vi "ChuongTrinhLabVIEW.vi"() -> ()   [LabVIEW 2020]
uses:
  <vilib>/MakerHub/LINX/Public/Peripherals/Analog/Analog Read 1 Chan.vi
  <vilib>/MakerHub/LINX/Public/Peripherals/PWM/PWM Set Duty Cycle 1 Chan.vi
  <vilib>/MakerHub/LINX/Public/Peripherals/Analog/Analog Read N Chans.vi
  <vilib>/MakerHub/LINX/Private/Local IO/LinxAnalogRead.vi
  <vilib>/MakerHub/LINX/Public/Utilities/Check Channel.vi
  <vilib>/MakerHub/LINX/Public/Utilities/Open Serial.vi
  <vilib>/addons/control/pid/pid.llb/PID Gain Schedule (DBL).vi
  <vilib>/addons/control/pid/pid.llb/PID (DBL).vi
  <vilib>/MakerHub/LINX/Private/Utilties/Generate Error.vi
  <vilib>/MakerHub/LINX/Public/Peripherals/PWM/PWM Set Duty Cycle N Chans.vi
  <vilib>/MakerHub/LINX/LMH-LINX.lvlib
  <vilib>/addons/control/pid/NI_PID_pid.lvlib
panel:
  in  "Tab Control 3":enum32{"Page 1"}(tab)
  in  "Bang Thong So":string[][](table)
  out "Thong so":T1(graph)
  out "Cam bien khi gas":dbl
  out "nhiet do":dbl(slide) scale=0.0..100.0
  out "Do am":dbl(slide) scale=0.0..100.0
  out "?":dbl
  out "?":dbl
  out "CANH BAO MUA":string
  out "CANH BAO KHI GAS":string
  in  "Tab Control 2":enum32{"PID"}(tab)
  in  "PID gain schedule":T2(array[cluster])=[{"PID gains"={"proportional gain (Kc)"=1.0, "integral time (Ti, min)"=0.01, "derivative time (Td, min)"=0.0}, "max value"=100.0}] {"max value" format="%.2f"; "PID gains"."derivative time (Td, min)" format="%.3f"; "PID gains"."integral time (Ti, min)" format="%.3f"; "PID gains"."proportional gain (Kc)" format="%.3f"}
  out "PID":T3(graph)
  in  "Set point":dbl
  in  "Tab Control":enum32{"Control"}(tab)
  in  "livingRoom":bool
  in  "Control DOOR":bool
  out "State Door":string
  in  "BedRoom":bool
  in  "kitchen":bool
  in  "Control Cua Cuon":bool
  in  "Control Dan Phoi":bool
  out "State Cua Cuon":string
  out "State Dan Phoi":string
  in  "Serial Port":refnum<visa-resource-name>="N/A"
  in  "?":bool
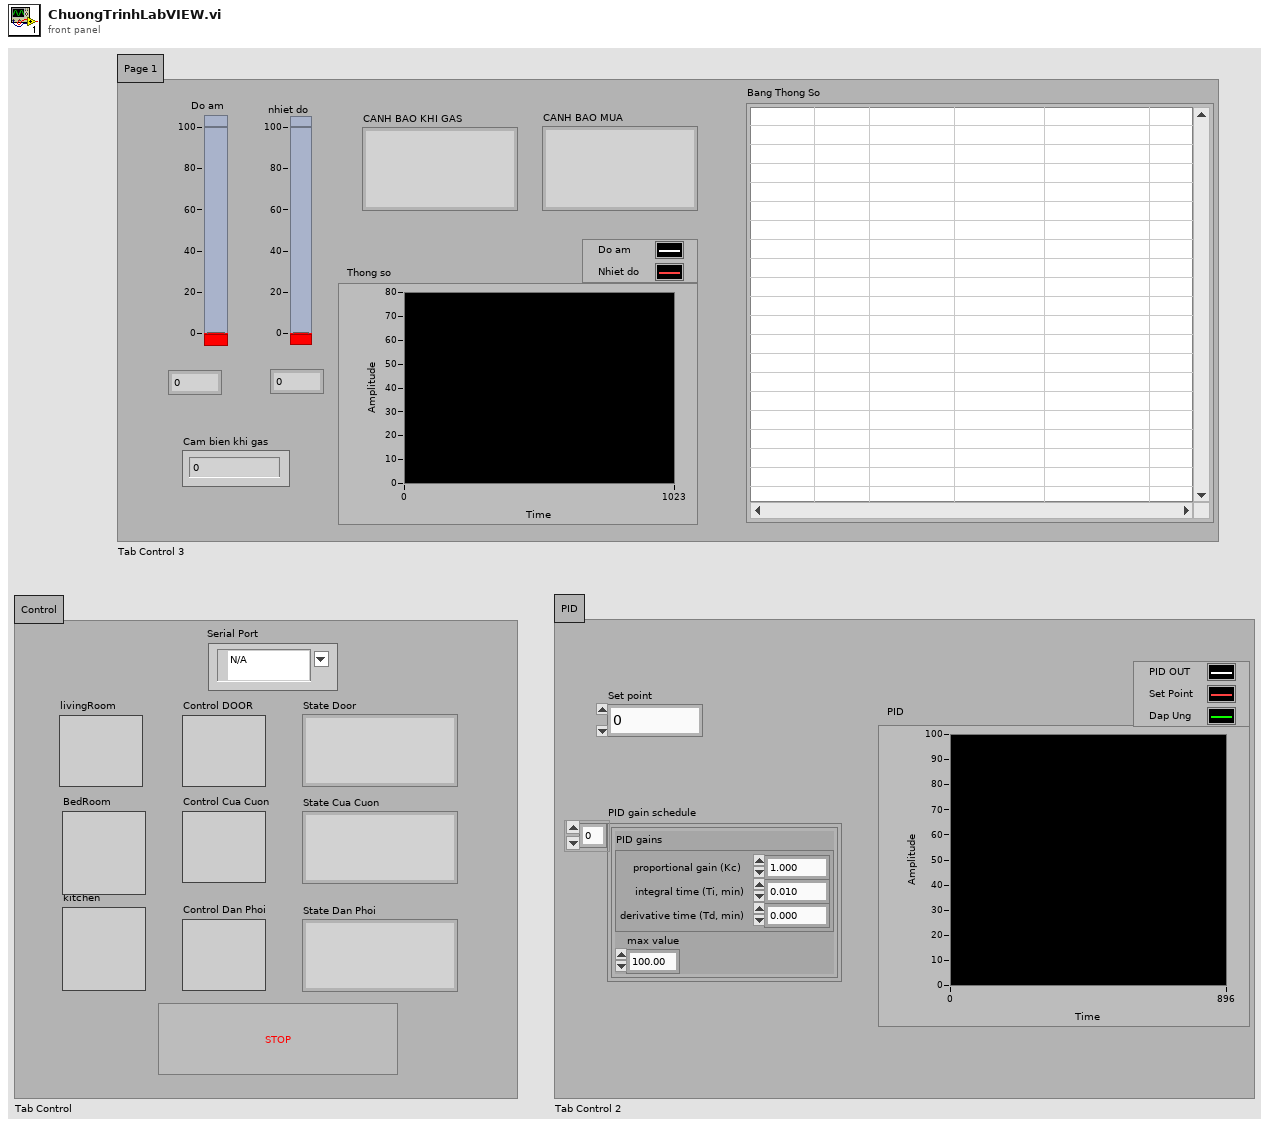
[diagram p1: front panel]
types:
  T1 = cluster{"Numeric Control":u8, "Numeric Control":u8}
  T2 = cluster{"PID gains":cluster{"proportional gain (Kc)":dbl, "integral time (Ti, min)":dbl, "derivative time (Td, min)":dbl}, "max value":dbl}[]
  T3 = cluster{"output":dbl, "Set point":dbl, "Numeric Control":u8}
  T4 = typedef "LMH-LINX.lvlib/LINX Ref.ctl" = cluster{"IO":T5, "Interface":T6, "LINX Device Config":T7}
  T5 = typedef "LMH-LINX.lvlib/Platform.ctl" = enum16{"Remote", "Local"}
  T6 = typedef "LMH-LINX.lvlib/Interface.ctl" = enum16{"Serial", "TCP"}
  T7 = typedef "LMH-LINX.lvlib/Device.lvlib/LINX Device Config.ctl" = cluster{"Interface":T6, "COM Port":refnum<visa-resource-name>, "TCP Configuration":T8, "Device Family":u8, "Device ID":u8, "Device Name":string, "TCP Ref":refnum<k5>, "Channels":T9}
  T8 = typedef "LMH-LINX.lvlib/Device.lvlib/TCP Config.ctl" = cluster{"IP Address":string, "Port":u16}
  T9 = typedef "LMH-LINX.lvlib/Channels.ctl" = cluster{"DI":u8[], "DO":u8[], "AI":u8[], "AO":u8[], "PWM":u8[], "QE":u8[], "UART":u8[], "I2C 2":u8[], "SPI":u8[], "CAN":u8[], "Servo":u8[], "AI Ref (V)":dbl, "AI Resolution (Bits)":u8, "AO Ref (V)":dbl, "AO Resolution (Bits)":u8}
  T10 = cluster{"proportional gain (Kc)":dbl, "integral time (Ti, min)":dbl, "derivative time (Td, min)":dbl}
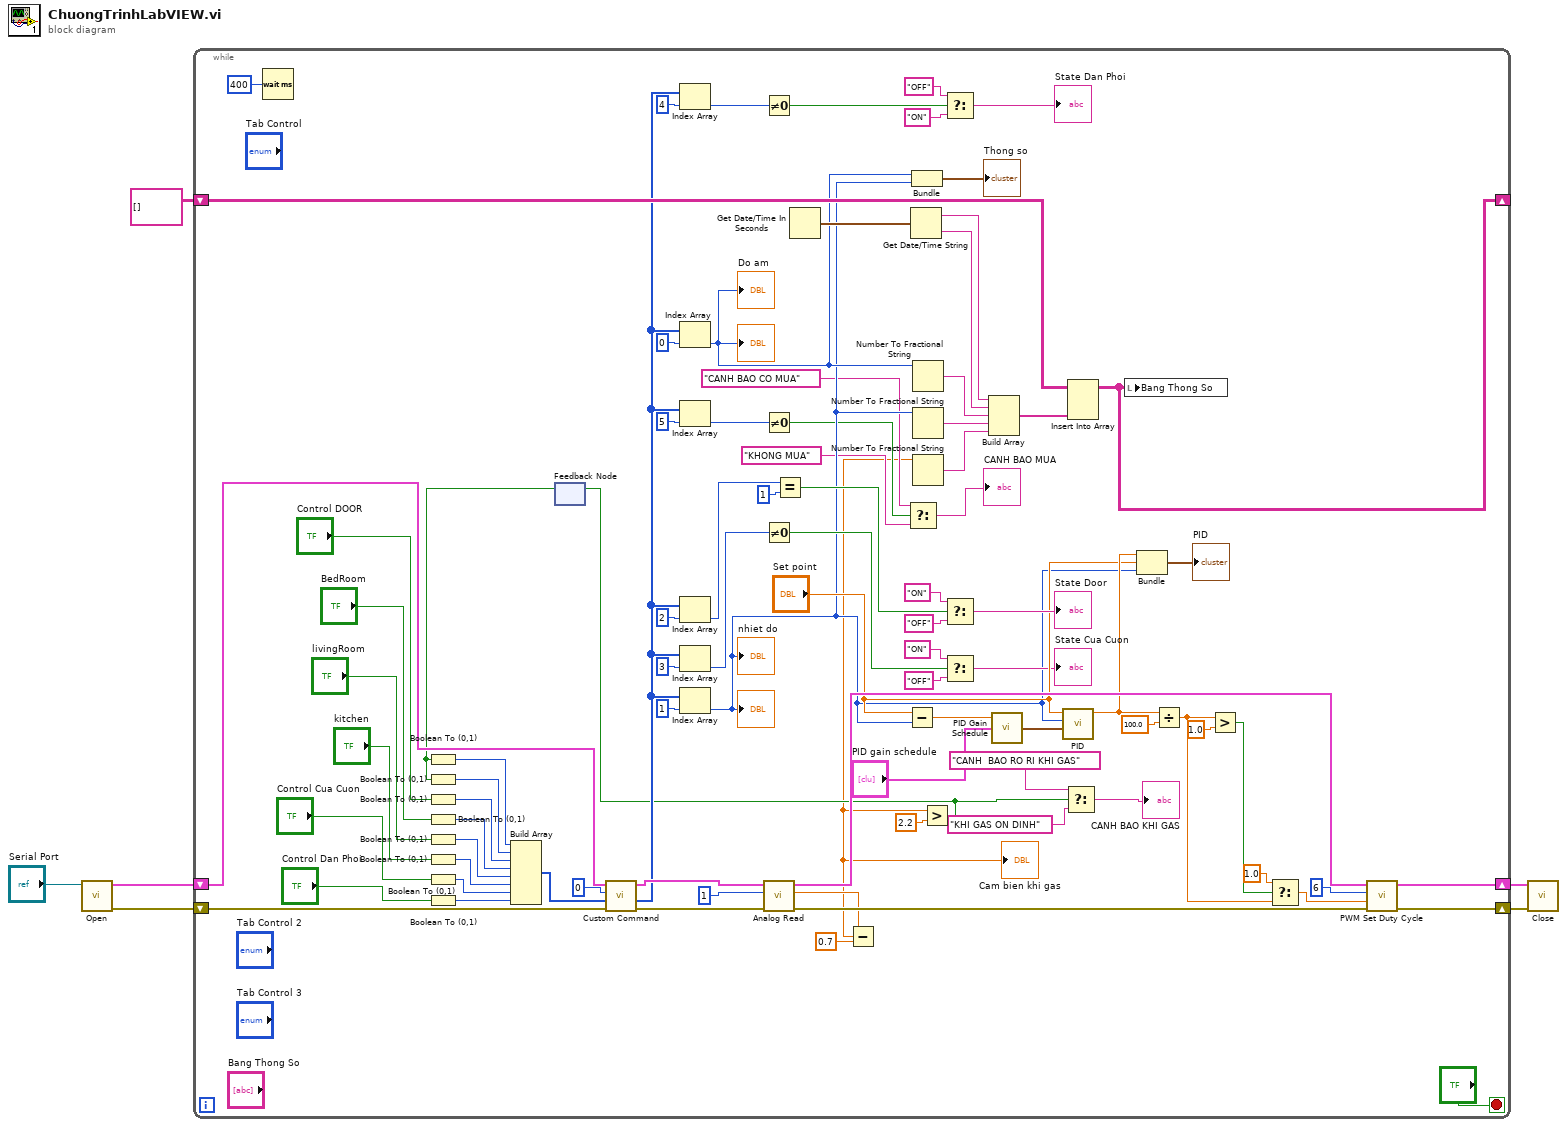
[diagram p0: block diagram]
diagram:
  n1 = call-poly <vilib>:"Open.vi"("Serial Port"="Serial Port") -> ("Error Out"=w4:errorcluster, "LINX Resource"=w6:T4)  [unwired: 8 in, 1 out]
  n2 = while {
    shift-right: [w46] -> w5
    shift-left: w6 -> [w94]
    shift-right: [w45] -> w3
    shift-left: w4 -> [w93]
    shift-right: [w52] -> _
    shift-left: string[][] [] -> [w53]
    stop <- "?" stop-if-true
    n3 = Wait (ms)(milliseconds to wait=u32 400) -> ()  [unwired: 1 out]
    n4 = Boolean To (0,1)(Boolean="Control DOOR") -> (0, 1=w83:i16)
    n5 = Boolean To (0,1)(Boolean="BedRoom") -> (0, 1=w73:i16)
    n6 = Boolean To (0,1)(Boolean="livingRoom") -> (0, 1=w69:i16)
    n7 = Boolean To (0,1)(Boolean="kitchen") -> (0, 1=w70:i16)
    n8 = Boolean To (0,1)(Boolean="Control Cua Cuon") -> (0, 1=w62:i16)
    n9 = Boolean To (0,1)(Boolean="Control Dan Phoi") -> (0, 1=w61:i16)
    n10 = feedback #1() -> (w56:bool)  [unwired: 1 in]
    n11 = Boolean To (0,1)(Boolean=w56) -> (0, 1=w88:i16)
    n12 = Boolean To (0,1)(Boolean=w56) -> (0, 1=w84:i16)
    n13 = Build Array(w88, w84, w83, w73, w69, w70, w62, w61) -> (w87:i16[])
    n14 = call <vilib>:"Custom Command.vi"("Error In"=w93, "Data"=w87, "Custom Command Number"=u16 0, "LINX Resource"=w94) -> ("Error Out"=w21:errorcluster, "Response"=w20:u8[], "LINX Resource"=w22:T4)  [unwired: 4 in, 1 out]
    n15 = Index Array(array=w20, index=4) -> (element=w65:u8)
    n16 = Index Array(array=w20, index=0) -> (element=w49:u8)
    "Do am" <- w49
    "?" <- w49
    n17 = Index Array(array=w20, index=5) -> (element=w18:u8)
    n18 = Index Array(array=w20, index=2) -> (element=w80:u8)
    n19 = Index Array(array=w20, index=3) -> (element=w66:u8)
    n20 = Index Array(array=w20, index=1) -> (element=w23:u8)
    "nhiet do" <- w23
    "?" <- w23
    n21 = Not Equal To 0?(x=w65) -> (x != 0?=w31:bool)
    n22 = Not Equal To 0?(x=w18) -> (x != 0?=w15:bool)
    n23 = Not Equal To 0?(x=w66) -> (x != 0?=w35:bool)
    n24 = call-poly <vilib>:"Analog Read.vi"("Error In"=w21, "Analog Channel"=u8 1, "LINX Resource"=w22) -> ("Error Out"=w47:errorcluster, "Voltage"=w9:dbl, "LINX Resource"=w48:T4)  [unwired: 5 in, 1 out]
    n25 = Equal?(x=w80, y=u8 1) -> (x = y?=w78:bool)
    n26 = Get Date/Time In Seconds() -> (seconds since 1Jan1904=w60:timestamp)
    n27 = Subtract(x=w9, y=0.7) -> (x-y=w7:dbl)
    "Cam bien khi gas" <- w7
    n28 = Subtract(x="Set point", y=w23) -> (x-y=w24:dbl)
    n29 = Select(t="CANH BAO CO MUA", s=w15, f="KHONG MUA") -> (s? t:f=→"CANH BAO MUA":string)
    n30 = Get Date/Time String(seconds (now)=w60) -> (date string=w59:string, time string=w58:string)  [unwired: 2 in]
    n31 = Bundle("Numeric Control"=w49, "Numeric Control"=w23) -> (→"Thong so":T1)  [unwired: 1 in]
    n32 = Number To Fractional String(number=w49) -> (F-format string=w57:string)  [unwired: 3 in]
    n33 = Number To Fractional String(number=w23) -> (F-format string=w55:string)  [unwired: 3 in]
    n34 = Number To Fractional String(number=w7) -> (F-format string=w51:string)  [unwired: 3 in]
    n35 = Greater?(x=w7, y=2.2) -> (0:w12:bool)
    n36 = feedback-in #1(w12) -> ()
    n37 = Select(t="OFF", s=w31, f="ON") -> (s? t:f=→"State Dan Phoi":string)
    n38 = Select(t="ON", s=w78, f="OFF") -> (s? t:f=→"State Door":string)
    n39 = Select(t="ON", s=w35, f="OFF") -> (s? t:f=→"State Cua Cuon":string)
    n40 = Build Array(w59, w58, w57, w55, w51) -> (w54:string[])
    n41 = call-poly <vilib>:"PID Gain Schedule.vi"("PID gain schedule"="PID gain schedule", "gain scheduling value"=w24) -> ("PID gains out"=w43:T10)  [unwired: 2 in, 1 out]
    n42 = call-poly <vilib>:"PID.vi"("PID gains"=w43, "process variable"=w23, "setpoint"="Set point") -> ("output"=w40:dbl)  [unwired: 7 in, 1 out]
    n43 = Select(t="CANH  BAO RO RI KHI GAS", s=w12, f="KHI GAS ON DINH") -> (s? t:f=→"CANH BAO KHI GAS":string)
    n44 = Insert Into Array(array=w53, new element=w54) -> (w52:string[][])  [unwired: 2 in]
    n45 = local write "Bang Thong So"(w52) -> ()
    n46 = Bundle("output"=w40, "Set point"="Set point", "Numeric Control"=w23) -> (→"PID":T3)  [unwired: 1 in]
    n47 = Divide(x=w40, y=100.0) -> (x/y=w26:dbl)
    n48 = Greater?(x=w26, y=1.0) -> (0:w28:bool)
    n49 = Select(t=1.0, s=w28, f=w26) -> (s? t:f=w25:dbl)
    n50 = call-poly <vilib>:"PWM Set Duty Cycle.vi"("Error In"=w47, "Duty Cycle (0-1)"=w25, "PWM Channel"=u8 6, "LINX Resource"=w48) -> ("Error Out"=w45:errorcluster, "LINX Resource"=w46:T4)  [unwired: 6 in]
  }
  n51 = call <vilib>:"Close.vi"("Error In"=w3, "LINX Resource"=w5) -> ()  [unwired: 9 in, 1 out]
